vi "Set Window GWL_Style.vi"(8 "error in (no error)":errorcluster, 10 "Style":u32, 11 "Hwnd":u32) -> (0 "error out":errorcluster)   [LabVIEW 2011]
doc: "This VI will set the window <B>Hwnd</B> GWL_Style."
uses:
  user32.dll
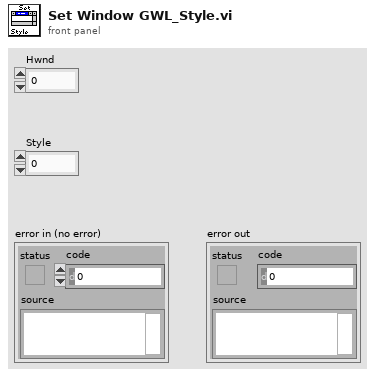
[diagram p1: front panel]
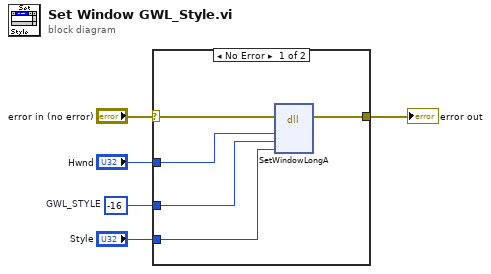
[diagram p0: block diagram]
diagram:
  w5 = -16  # GWL_STYLE
  n1 = case shown="No Error" "error in (no error)" {
    selector: "error in (no error)" -> [w8 w11]
    tunnel: w5 -> [w10 _]
    tunnel: "Hwnd" -> [w9 _]
    tunnel: [w7 w11] -> w3
    tunnel: "Style" -> [w6 _]
    frame No Error {
      n2 = dll-call lib="user32.dll" fn="SetWindowLongA" ("SetParent")(error in=w8, "Hwnd"=w9, "Index"=w10, "NewLong"=w6) -> (error out=w7:errorcluster)  [unwired: 6 in, 1 out]
    }
    frame Error {
    }
  }
  "error out" <- w3
